vi "Prepare WebSocket Stream.vi"(8 "error in (no error)":errorcluster, 11 "GodotServer in":refnum<class "GodotServer.lvclass">) -> (0 "error out":errorcluster, 2 "WebsocketStream":refnum<class "WebsocketStream.lvclass">, 3 "GodotServer out":refnum<class "GodotServer.lvclass">)   [LabVIEW 2020, in "GodotLV.lvlib" / "GodotServer.lvclass"]
uses:
  GodotServer.lvclass
  lv-stream-websocket/Stream-Websocket/Websocket Server/Websocket Server.lvclass
  lv-stream-websocket/Stream-Websocket/WebsocketStream/WebsocketStream.lvclass
  lv-stream-websocket/Stream-Websocket/Websocket Client/Websocket Client.lvclass
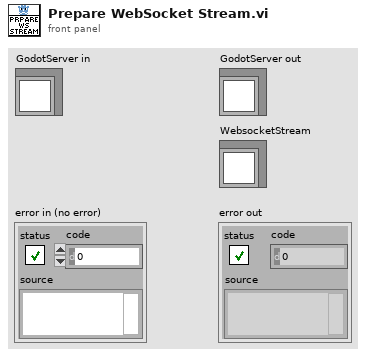
[diagram p1: front panel]
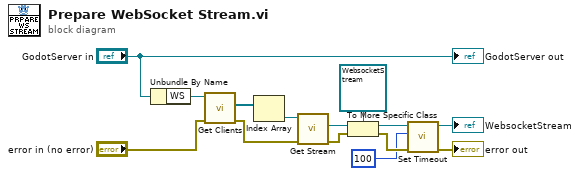
[diagram p0: block diagram]
diagram:
  n1 = Unbundle By Name("GodotServer in") -> ("WS"=w12:refnum<class "Websocket Server.lvclass">)
  n2 = call "Get Clients.vi"("error in (no error)"="error in (no error)", "Websocket Server in"=w12) -> ("error out"=w11:errorcluster, "Clients"=w14:refnum<class "Websocket Client.lvclass">[])  [unwired: 7 in, 1 out]
  n3 = Index Array(array=w14) -> (element=w13:refnum<class "Websocket Client.lvclass">)  [unwired: 1 in]
  n4 = call-dynamic "Get Stream.vi"("error in (no error)"=w11, "Websocket Client in"=w13) -> ("error out"=w5:errorcluster, "Stream"=w6:refnum<class "Stream.lvclass">)  [unwired: 7 in, 1 out]
  n5 = To More Specific Class(target class=refnum<class "WebsocketStream.lvclass"> refnum ("WebsocketStream in"), reference=w6, error in=w5) -> (specific class reference=w8:refnum<class "WebsocketStream.lvclass">, error out=w10:errorcluster)
  n6 = call "Set Timeout.vi"("error in (no error)"=w10, "Timeout ms"=100, "WebsocketStream in"=w8) -> ("error out"=→"error out":errorcluster, "WebsocketStream out"=→"WebsocketStream":refnum<class "WebsocketStream.lvclass">)  [unwired: 7 in]
  "GodotServer out" <- "GodotServer in"
